vi "Set X-Y ROI.vi"(8 "error in (no error)":errorcluster, 9 "ROI X":cluster{"Index":u32, "Length":u32}, 10 "ROI Y":cluster{"Index":u32, "Length":u32}, 11 "TG Base Graph in":refnum<class "TG Base Graph.lvclass">) -> (0 "error out":errorcluster, 3 "TG Base Graph out":refnum<class "TG Base Graph.lvclass">)   [LabVIEW 2023, in "TG Base Graph.lvclass"]
uses:
  TG Base Graph.lvclass
  TG Base Graph.lvclass/TG Base Graph.ctl
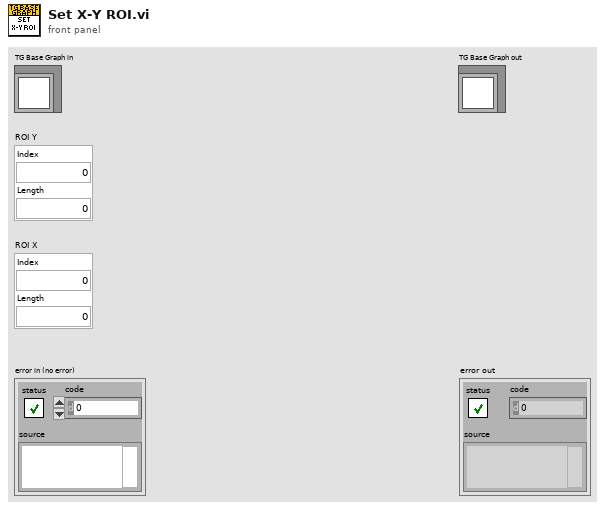
[diagram p1: front panel]
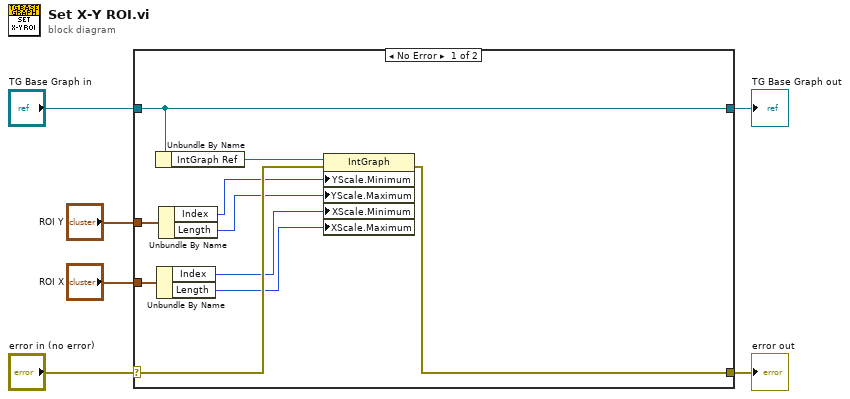
[diagram p0: block diagram]
diagram:
  n1 = case shown="No Error" "error in (no error)" {
    selector: "error in (no error)" -> [w14 w18]
    tunnel: [w7 w18] -> w5
    tunnel: [w16 w17] -> w3
    tunnel: "TG Base Graph in" -> [w16 w17]
    tunnel: "ROI Y" -> [w13 _]
    tunnel: "ROI X" -> [w10 _]
    frame No Error {
      n2 = Unbundle By Name(w16) -> ("IntGraph Ref"=w15:refnum<vi>)
      n3 = Unbundle By Name(w10) -> ("Index"=w9:u32, "Length"=w8:u32)
      n4 = Unbundle By Name(w13) -> ("Index"=w12:u32, "Length"=w11:u32)
      n5 = property class="IntGraph"(reference=w15, error in=w14, "YScale.Minimum"=w12, "YScale.Maximum"=w11, "XScale.Minimum"=w9, "XScale.Maximum"=w8) -> (error out=w7:errorcluster)  [unwired: 1 out]
    }
    frame Error {
    }
  }
  "error out" <- w5
  "TG Base Graph out" <- w3
